vi "get HovaCAL Komponente fix Gasnummer Auswahl.vi"(9 "AutoLin MFC in":u16, 10 "MFV Komponente fix in":u16[](array[numeric]), 11 "Gasnummer EPA":T1 min=1 max=5) -> (3 "MFV Komponente fix out":u16)   [LabVIEW 2020, in "Linearisierung v2.lvlib" / "Gasteiler.lvlib" / "HovaCAL_Interface.lvlib" / "Helper.lvlib"]
uses:
  Helper.lvlib
  Gasnumber.ctl
  Linearisierung v2.lvlib
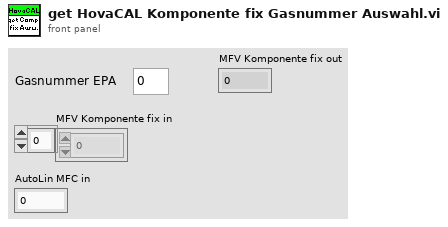
[diagram p1: front panel]
types:
  T1 = typedef "Linearisierung v2.lvlib/Gasnumber.ctl" = u8
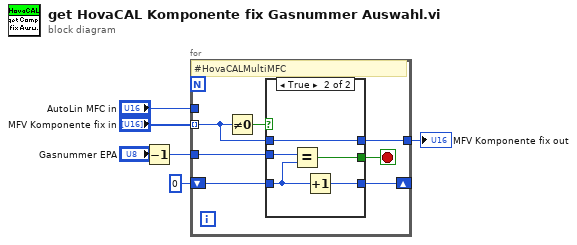
[diagram p0: block diagram]
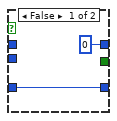
[diagram p2: hidden frame]
diagram:
  n1 = Decrement(x="Gasnummer EPA") -> (x-1=w1:T1)
  n2 = for {
    tunnel: w1 -> [w10]
    tunnel: "MFV Komponente fix in" -> [w9] mode=indexing
    tunnel: "AutoLin MFC in" -> [_]
    shift-right: [w12] -> _
    shift-left: 0 -> [w11]
    tunnel: [w8] -> w2
    stop <- w7 stop-if-true
    # "#HovaCALMultiMFC"
    n3 = Not Equal To 0?(x=w9) -> (x != 0?=w13:bool)
    n4 = case shown="True" w13 {
      tunnel: w11 -> [w15 w18]
      tunnel: [w15 w20] -> w12
      tunnel: w10 -> [_ w19]
      tunnel: w9 -> [_ w17]
      tunnel: [u16 0 ("MFV Komponente fix") w17] -> w8
      tunnel: [_ w16] -> w7
      frame False {
      }
      frame True {
        n5 = Equal?(x=w19, y=w18) -> (x = y?=w16:bool)
        n6 = Increment(x=w18) -> (x+1=w20:i32)
      }
    }
  }
  "MFV Komponente fix out" <- w2
